vi "testNull.vi"(8 "error in (no error)":errorcluster, 11 "TestCase in":refnum<class "JsonTest.lvclass">) -> (0 "error out":errorcluster, 3 "TestCase out":refnum<class "JsonTest.lvclass">)   [LabVIEW 2017]
uses:
  JsonTest.lvclass
  <vilib>/addons/_JKI Toolkits/VI Tester/TestCase.llb/TestCase.lvclass
  Source/Variant JSON API.lvlib
  C:/Program Files (x86)/National Instruments/LabVIEW 2017/vi.lib/addons/_JKI Toolkits/VI Tester/TestCase.llb/TestCase.lvclass
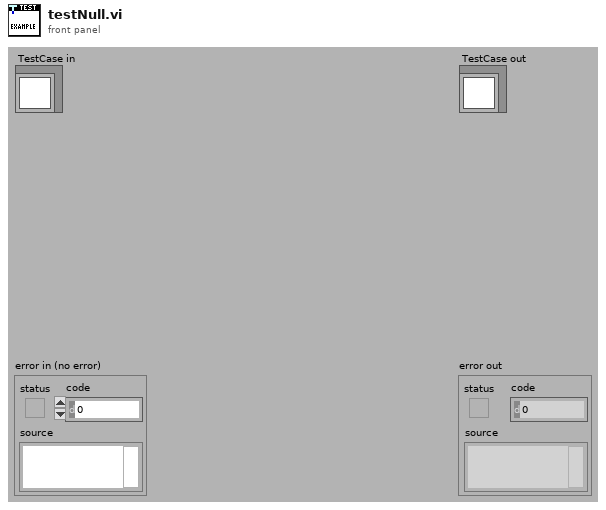
[diagram p1: front panel]
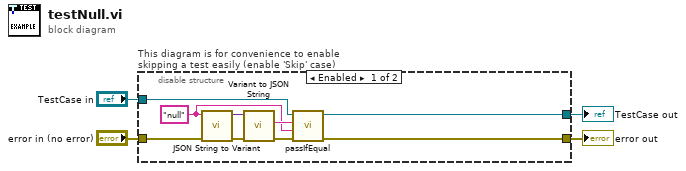
[diagram p0: block diagram]
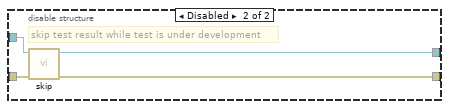
[diagram p2: hidden frame]
diagram:
  n1 = disable-structure "This diagram is for convenience to enable skipping a test easily (enable 'Skip' case)" shown="Enabled" {
    disable-tunnel: "TestCase in" -> [w12 w17]
    disable-tunnel: [w11 w15] -> w1
    disable-tunnel: [w13 w16] -> w3
    disable-tunnel: "error in (no error)" -> [w7 w14]
    frame Enabled {
      w8 = "null" ("JSON String")
      n2 = call "JSON String to Variant.vi"("error in (no error)"=w7, "JSON String"=w8) -> ("error out"=w6:errorcluster, "Variant out"=w10:variant)  [unwired: 8 in]
      n3 = call "Variant to JSON String.vi"("error in (no error)"=w6, "Variant in"=w10) -> ("error out"=w5:errorcluster, "String"=w9:string)  [unwired: 7 in, 1 out]
      n4 = call-dynamic "passIfEqual.vi"("error in (no error)"=w5, "y"=w8, "x"=w9, "TestCase in"=w12) -> ("error out"=w13:errorcluster, "TestCase out"=w11:refnum<class "JsonTest.lvclass">)  [unwired: 6 in]
    }
    frame Disabled {
      # "skip test result while test is under development"
      n5 = call <vilib>:"skip.vi"("error in (no error)"=w14, "TestCase in"=w17) -> ("error out"=w16:errorcluster, "TestCase out"=w15:refnum<class "JsonTest.lvclass">)  [unwired: 8 in]
    }
  }
  "error out" <- w3
  "TestCase out" <- w1
